vi "PWM2 Start.vi"(9 "RunTimeUs":u32, 10 "ChannelIndex":u8, 11 "DevHandle":i32) -> (3 "function return":i32)   [LabVIEW 2010, in "usb2pwm.lvlib"]
doc: "int WINAPI PWM2_Start(int DevHandle, unsigned char ChannelIndex, unsigned int RunTimeUs);"
uses:
  usb2pwm.lvlib
  USB2XXX/trunk/USB2XXX/USB2XXX/vs2019/Release/USB2XXX.dll
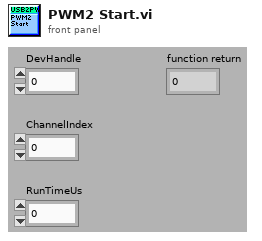
[diagram p1: front panel]
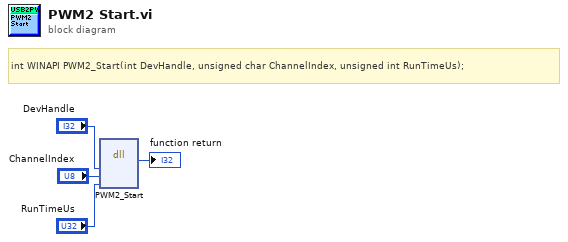
[diagram p0: block diagram]
diagram:
  # "int WINAPI PWM2_Start(int DevHandle, unsigned char ChannelIndex, unsigned int RunTimeUs);"
  n1 = dll-call lib="E:/Projects/USB2XXX/trunk/USB2XXX/USB2XXX/vs2019/Release/USB2XXX.*" fn="PWM2_Start"("DevHandle"="DevHandle", "ChannelIndex"="ChannelIndex", "RunTimeUs"="RunTimeUs") -> (→"function return":i32)  [unwired: 6 in, 2 out]
